vi "CANopen Write RPDO.vi"() -> ()   [LabVIEW 2016]
doc: "This example demonstrates how to write CANopen RPDO data to the device."
uses:
  <vilib>/userdefined/High Color/nirio_resource_hc.ctl
  <vilib>/Platform/TimedLoop/XDataNode/timing_clust.ctl
  <vilib>/Platform/TimedLoop/XDataNode/nitl_modes.ctl
  <vilib>/Platform/TimedLoop/XDataNode/wakeup.ctl
  <vilib>/FPGAPlugInAG/cRIO-9033/niLvFpga_Open_cRIO-9033.vi
  <vilib>/rvi/interface/common/dynamic/niFpgaDynamicAddResources.vi
  <vilib>/CANopenLib/CANOPEN.llb/CANopen Interface Create.vi
  <vilib>/CANopenLib/CANOPEN.llb/CANopen RPDO Create.vi
  <vilib>/CANopenLib/CANOPEN.llb/CANopen RPDO Start.vi
  <vilib>/CANopenLib/CANOPEN.llb/CANopen RPDO Close.vi
  <vilib>/CANopenLib/CANOPEN.llb/CANopen Interface Close.vi
  <vilib>/FPGAPlugInAG/Dynamic/niLvFpga_Close_Dynamic.vi
  <vilib>/rvi/interface/nirviOpenFPGA/nirviOpenFPGA.xnode
  Users/s163601/Desktop/05-28/FPGA Bitfiles/project_FPGATarget_MainFPGA_S9ZLErdeBuw.lvbitx
  Users/s163601/Desktop/05-28/RT/FPGA/MainFPGA.vi
  <vilib>/Platform/TimedLoop/XDataNode/XDataNode.xnode
  <vilib>/rvi/interface/nirviCloseFPGA/nirviCloseFPGA.xnode
  <resource>/objmgr/CANopenPDO.rc
  <vilib>/Platform/TimedLoop/XDataNode/XDNodeRunTimeDep.lvlib
panel:
  in  "error in":errorcluster
  in  "RPDO data":u8[](array[numeric])=[0, 0, 0, 0, 0, 0, 0, 0]
  in  "period (ms)":i64=10
  in  "stop":bool
  in  "auto start":bool
  in  "event time":u8=10
  in  "inhibit time":u8=10
  in  "node-ID":u8=1 min=1 max=127 step=1
  in  "PDO channel":u8(ring) items=["PDO 1", "PDO 2", "PDO 3", "PDO 4"]
  in  "baud rate":u32(ring)=2 items=["1 Mbit/s"=0, "800 kbit/s"=1, "500 kbit/s"=2, "250 kbit/s"=3, "125 kbit/s"=4, "50 kbit/s"=6, "20 kbit/s"=7, "10 kbit/s"=8]
  in  "CANopen interface":u32(ring) items=["CANopen01", "CANopen02", "CANopen03", "CANopen04", "CANopen05", "CANopen06", "CANopen07", "CANopen08", "CANopen09", "CANopen10", "CANopen11", "CANopen12", "CANopen13", "CANopen14", "CANopen15", "CANopen16", "CANopen17", "CANopen18", "CANopen19", "CANopen20", "CANopen21", "CANopen22", "CANopen23", "CANopen24", "CANopen25", "CANopen26", "CANopen27", "CANopen28", "CANopen29", "CANopen30", "CANopen31", "CANopen32"]
  # "Overview: This example demonstrates how to write CANopen RPDO data to the device.\nRequirements: Connect CANopen module with a slave device. \nInstructions:\n1. Specify the values of CANopen interface, baud rate of the CANopen interface and node-ID of the slave device.\n2. Run this VI.\n3. Click STOP to stop the VI."
  # "Create CANopen interface and RPDO object"
  # "Set RPDO properties"
  # "Write RPDO data"
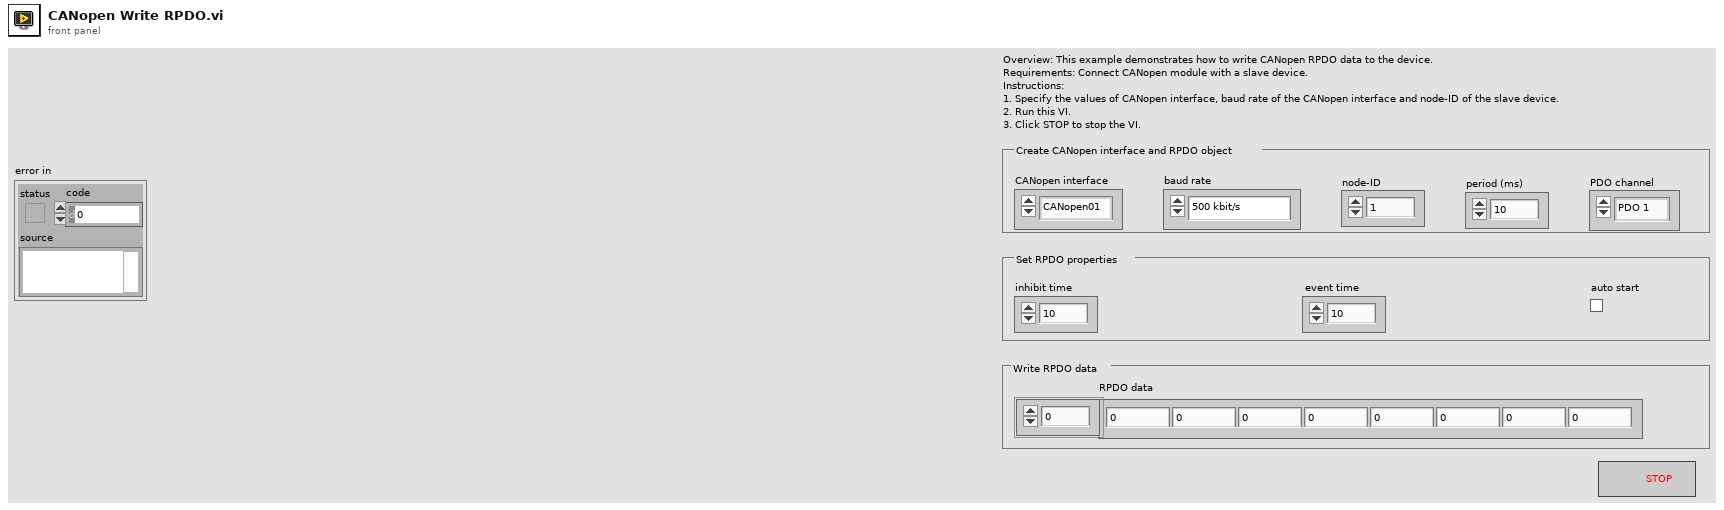
[diagram p1: front panel]
types:
  T1 = typedef "nirio_resource_hc.ctl" = tag
  T2 = typedef "XDNodeRunTimeDep.lvlib/timing_clust.ctl" = cluster{"Expected End [f-1]":u64, "Actual End [f-1]":u64, "Finished Late? [f-1]":bool, "Expected End [i-1]":u64, "Actual End [i-1]":u64, "Finished Late? [i-1]":bool, "Expected Start [i]":u64, "Actual Start [i]":u64, "Expected Start [f]":u64, "Actual Start [f]":u64, "Source Name":string, "Structure Name":string, "Period":i64, "Deadline":i64, "Offset":i64, "Start":i64, "Priority":i32, "Timeout":i32, "Mode":T3, "Wakeup Reason":T4, "Error":errorcluster, "Source Type":string, "Secondary Source Type":string, "Global End Time":u64, "Global Start Time":u64, "Frame Duration":u64, "Iteration Duration":u64, "Assigned CPU":i32, "I/O Scan Engine Mode":u32}
  T3 = typedef "XDNodeRunTimeDep.lvlib/nitl_modes.ctl" = enum32{"No Change", "Process missed periods, maintain original phase", "Discard missed periods, maintain original phase", "Process missed periods, ignore original phase", "Discard missed periods, ignore original phase"}
  T4 = typedef "XDNodeRunTimeDep.lvlib/wakeup.ctl" = enum32{"Normal", "Aborted", "Asynchronous wakeup", "Timing source error", "Timed loop error", "Timeout"}
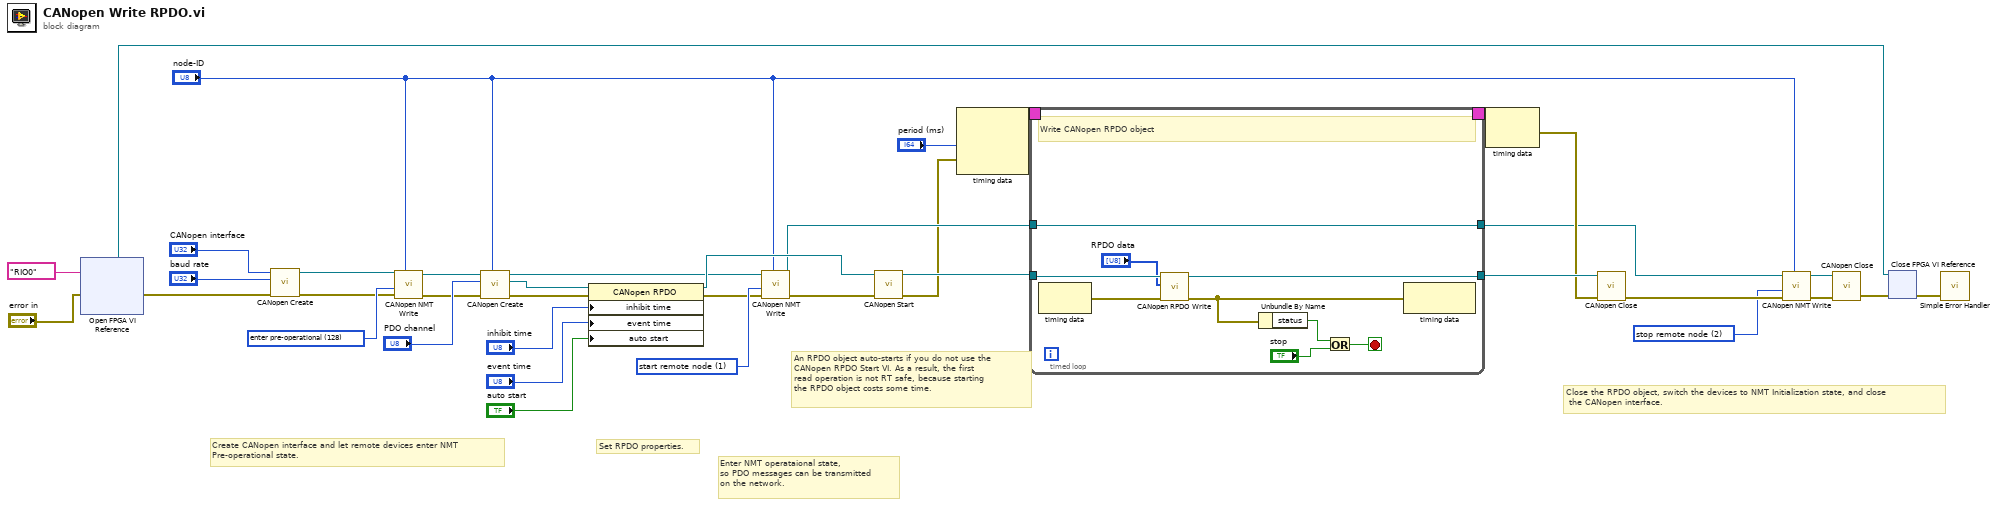
[diagram p0: block diagram]
diagram:
  w15 = u16 1 items=["start remote node"=1, "stop remote node"=2, "enter pre-operational"=128, "reset node"=129, "reset communication"=130] ("command")
  w17 = u16 2 items=["start remote node"=1, "stop remote node"=2, "enter pre-operational"=128, "reset node"=129, "reset communication"=130] ("command")
  w30 = u16 128 items=["start remote node"=1, "stop remote node"=2, "enter pre-operational"=128, "reset node"=129, "reset communication"=130] ("command")
  # "An RPDO object auto-starts if you do not use the \nCANopen RPDO Start VI. As a result, the first \nread operation is not RT safe, because starting \nthe RPDO object costs some time."
  # "Close the RPDO object, switch the devices to NMT Initialization state, and close\n the CANopen interface."
  # "Create CANopen interface and let remote devices enter NMT\nPre-operational state."
  # "Set RPDO properties."
  # "Enter NMT operataional state,\nso PDO messages can be transmitted\non the network."
  n1 = xnode ("Open FPGA VI Reference")("error in"="error in", "resource name"=T1 "RIO0") -> ("FPGA VI Reference Out"=w1:refnum<k20>, "error out"=w4:errorcluster)
  n2 = call-poly <vilib>:"CANopen Create.vi"("error in (no error)"=w4, "baud rate"="baud rate", "interface name"="CANopen interface") -> ("error out"=w29:errorcluster, "interface object out"=w28:refnum<k20>)  [unwired: 7 in]
  n3 = call <vilib>:"CANopen NMT Write.vi"("node-ID (0)"="node-ID", "error in (no error)"=w29, "command"=w30, "interface object in"=w28) -> ("error out"=w24:errorcluster, "interface object out"=w34:refnum<k20>)  [unwired: 6 in]
  n4 = call-poly <vilib>:"CANopen Create.vi"("node-ID"="node-ID", "error in (no error)"=w24, "PDO channel"="PDO channel", "interface object in"=w34) -> ("error out"=w25:errorcluster, "RPDO object out"=w27:refnum<k20>, "interface object out"=w14:refnum<k20>)  [unwired: 5 in]
  n5 = property class="CANopen RPDO"(reference=w27, error in=w25, "inhibit time"="inhibit time", "event time"="event time", "auto start"="auto start") -> (reference out=w26:refnum<k20>, error out=w12:errorcluster)
  n6 = call <vilib>:"CANopen NMT Write.vi"("node-ID (0)"="node-ID", "error in (no error)"=w12, "command"=w15, "interface object in"=w14) -> ("error out"=w11:errorcluster, "interface object out"=w13:refnum<k20>)  [unwired: 6 in]
  n7 = call-poly <vilib>:"CANopen Start.vi"("error in (no error)"=w11, "RPDO object in"=w26) -> ("error out"=w10:errorcluster, "RPDO object out"=w31:refnum<k20>)  [unwired: 8 in]
  n8 = node-c288("period (ms)", w10) -> (w38:T2)  [unwired: 1 in]
  n9 = timed-loop {
    tunnel: [w47] -> w33
    tunnel: w31 -> [w46]
    timing: w38 -> [_]
    timing-out: [_] -> w37
    tunnel: w13 -> [w45]
    tunnel: [w45] -> w7
    stop <- w44 stop-if-true
    # "Write CANopen RPDO object"
    n10 = node-c288() -> (w41:errorcluster)  [unwired: 1 in]
    n11 = call <vilib>:"CANopen RPDO Write.vi"("error in (no error)"=w41, "data"="RPDO data", "RPDO object in"=w46) -> ("error out"=w40:errorcluster, "RPDO object out"=w47:refnum<k20>)  [unwired: 7 in]
    n12 = Unbundle By Name(w40) -> ("status"=w42:bool)
    n13 = Or(x=w42, y="stop") -> (x .or. y?=w44:bool)
    n14 = node-c288(w40) -> ()  [unwired: 1 out]
  }
  n15 = node-c288(w37) -> (w9:errorcluster)
  n16 = call-poly <vilib>:"CANopen Close.vi"("error in (no error)"=w9, "RPDO object in"=w33) -> ("error out"=w20:errorcluster)  [unwired: 9 in]
  n17 = call <vilib>:"CANopen NMT Write.vi"("node-ID (0)"="node-ID", "error in (no error)"=w20, "command"=w17, "interface object in"=w7) -> ("error out"=w19:errorcluster, "interface object out"=w18:refnum<k20>)  [unwired: 6 in]
  n18 = call-poly <vilib>:"CANopen Close.vi"("error in (no error)"=w19, "interface object in"=w18) -> ("error out"=w3:errorcluster)  [unwired: 9 in]
  n19 = xnode "Close FPGA VI Reference"("FPGA VI Reference In"=w1, "error in"=w3) -> ("error out"=w2:errorcluster)
  n20 = call <vilib>:"Simple Error Handler.vi"("error in (no error)"=w2) -> ()  [unwired: 4 in, 5 out]
